vi "Stability Analysis module.vi"(1 "Step Zero":bool, 2 "Step":i32, 3 "PercentIn":dbl, 4 "Input":dbl) -> (0 "Parameter Stable?":bool)   [LabVIEW 2018]
panel:
  out "STCount":dbl
  out "PercentOut":dbl
  out "Numeric 4":dbl
  out "Numeric 3":dbl
  out "Numeric 2":dbl
  out "Numeric 1":dbl
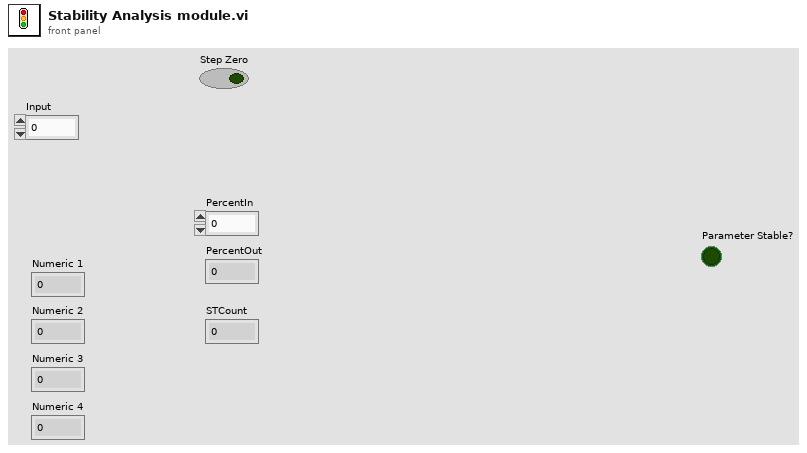
[diagram p1: front panel]
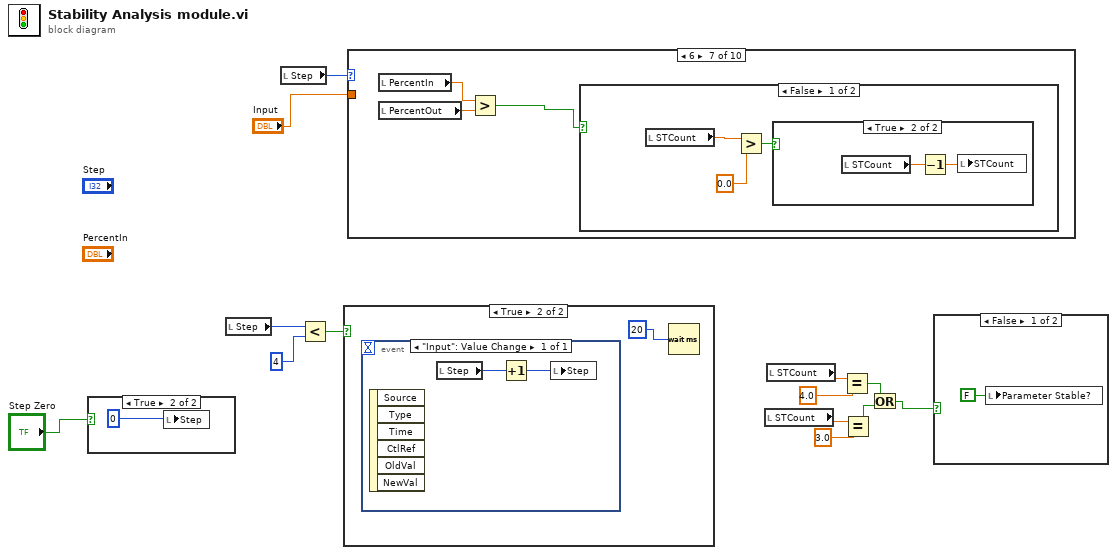
[diagram p0: block diagram]
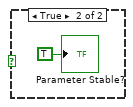
[diagram p3: hidden frame]
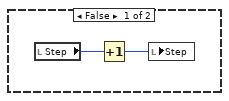
[diagram p4: hidden frame]
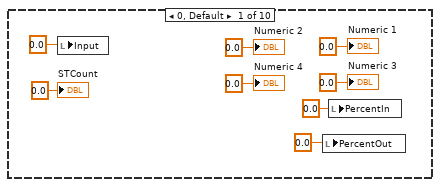
[diagram p5: hidden frame]
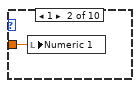
[diagram p6: hidden frame]
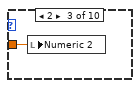
[diagram p7: hidden frame]
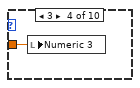
[diagram p8: hidden frame]
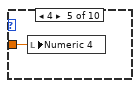
[diagram p9: hidden frame]
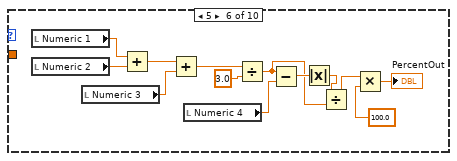
[diagram p10: hidden frame]
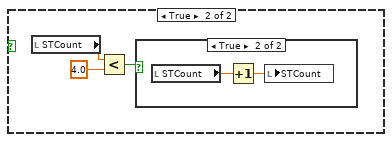
[diagram p12: hidden frame]
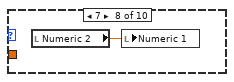
[diagram p14: hidden frame]
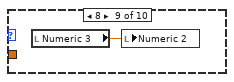
[diagram p15: hidden frame]
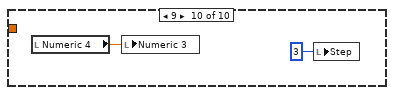
[diagram p16: hidden frame]
diagram:
  n1 = case shown="True" "Step Zero" {
    frame False {
    }
    frame True {
      n2 = local write "Step"(0 ("Step Go")) -> ()
    }
  }
  n3 = local read "Step"() -> (w10:i32)
  n4 = local read "Step"() -> (w12:i32)
  n5 = Less?(x=w10, y=4) -> (x < y?=w11:bool)
  n6 = case shown="True" w11 {
    frame False {
      n7 = local read "Step"() -> (w16:i32)
      n8 = Increment(x=w16) -> (x+1=w15:i32)
      n9 = local write "Step"(w15) -> ()
    }
    frame True {
      n10 = event shown="[0] \"Input\": Value Change" {
        selector: _ -> [_]
        dyn-events: _ -> [_]
        timeout: _ -> [_]
        event "Input": Value Change {
          n11 = event-data() -> ()  [unwired: 1 in, 6 out]
          n12 = local read "Step"() -> (w19:i32)
          n13 = Increment(x=w19) -> (x+1=w18:i32)
          n14 = local write "Step"(w18) -> ()
        }
      }
      n15 = Wait (ms)(milliseconds to wait=u32 20) -> ()  [unwired: 1 out]
    }
  }
  n16 = case shown="6" w12 {
    tunnel: "Input" -> [_ w28 w29 w30 w31 _ _ _ _ _]
    frame 0, Default {
      n17 = local write "Input"(0.0 ("Input")) -> ()
      n18 = local write "PercentOut"(0.0 ("Numeric")) -> ()
      n19 = local write "PercentIn"(0.0 ("PercentIn")) -> ()
      "Numeric 1" <- 0.0 ("Numeric 1")
      "Numeric 3" <- 0.0 ("Numeric 3")
      "Numeric 2" <- 0.0 ("Numeric 2")
      "Numeric 4" <- 0.0 ("Numeric 4")
      "STCount" <- 0.0 ("STCount")
    }
    frame 1 {
      n20 = local write "Numeric 1"(w28) -> ()
    }
    frame 2 {
      n21 = local write "Numeric 2"(w29) -> ()
    }
    frame 3 {
      n22 = local write "Numeric 3"(w30) -> ()
    }
    frame 4 {
      n23 = local write "Numeric 4"(w31) -> ()
    }
    frame 5 {
      n24 = local read "Numeric 1"() -> (w44:dbl)
      n25 = local read "Numeric 2"() -> (w43:dbl)
      n26 = local read "Numeric 3"() -> (w42:dbl)
      n27 = Add(x=w44, y=w43) -> (x+y=w41:dbl)
      n28 = Add(x=w41, y=w42) -> (x+y=w40:dbl)
      n29 = local read "Numeric 4"() -> (w36:dbl)
      n30 = Divide(x=w40, y=3.0) -> (x/y=w33:dbl)
      n31 = Subtract(x=w33, y=w36) -> (x-y=w35:dbl)
      n32 = Absolute Value(x=w35) -> (abs(x)=w34:dbl)
      n33 = Divide(x=w34, y=w33) -> (x/y=w32:dbl)
      n34 = Multiply(x=w32, y=100.0) -> (x*y=→"PercentOut":dbl)
    }
    frame 6 {
      n35 = local read "PercentIn"() -> (w47:dbl)
      n36 = local read "PercentOut"() -> (w46:dbl)
      n37 = Greater?(x=w47, y=w46) -> (0:w45:bool)
      n38 = case shown="False" w45 {
        frame False {
          n39 = local read "STCount"() -> (w49:dbl)
          n40 = Greater?(x=w49, y=0.0) -> (0:w50:bool)
          n41 = case shown="True" w50 {
            frame False {
            }
            frame True {
              n42 = local read "STCount"() -> (w52:dbl)
              n43 = Decrement(x=w52) -> (x-1=w51:dbl)
              n44 = local write "STCount"(w51) -> ()
            }
          }
        }
        frame True {
          n45 = local read "STCount"() -> (w53:dbl)
          n46 = Less?(x=w53, y=4.0) -> (x < y?=w55:bool)
          n47 = case shown="True" w55 {
            frame False {
            }
            frame True {
              n48 = local read "STCount"() -> (w56:dbl)
              n49 = Increment(x=w56) -> (x+1=w57:dbl)
              n50 = local write "STCount"(w57) -> ()
            }
          }
        }
      }
    }
    frame 7 {
      n51 = local read "Numeric 2"() -> (w58:dbl)
      n52 = local write "Numeric 1"(w58) -> ()
    }
    frame 8 {
      n53 = local read "Numeric 3"() -> (w59:dbl)
      n54 = local write "Numeric 2"(w59) -> ()
    }
    frame 9 {
      n55 = local read "Numeric 4"() -> (w61:dbl)
      n56 = local write "Numeric 3"(w61) -> ()
      n57 = local write "Step"(3 ("Step")) -> ()
    }
  }
  n58 = local read "STCount"() -> (w4:dbl)
  n59 = local read "STCount"() -> (w5:dbl)
  n60 = Equal?(x=w5, y=4.0) -> (x = y?=w8:bool)
  n61 = Equal?(x=w4, y=3.0) -> (x = y?=w7:bool)
  n62 = Or(x=w8, y=w7) -> (x .or. y?=w6:bool)
  n63 = case shown="False" w6 {
    frame False {
      n64 = local write "Parameter Stable?"(FALSE ("Parameter Stable?")) -> ()
    }
    frame True {
      "Parameter Stable?" <- TRUE ("Parameter Stable?")
    }
  }
